vi "LED Control Module Main.vi"(8 "error in":errorcluster) -> (0 "error out":errorcluster)   [LabVIEW 2018, in "LED Control Module.lvlib"]
uses:
  LED Control Module.lvlib
  Public Controls/LVS Settings.ctl
  Public Controls/LVS Limits.ctl
  Public Controls/LVS Instruments.ctl
  Public Controls/TestData.ctl
  INI/INI File Control.ctl
  Public Controls/LVS Testplan.ctl
  Private Controls/Module Data Cluster.ctl
  Private Controls/Module Action.ctl
  <vilib>/Utility/error.llb/DialogType.ctl
  Modules/Entry Console/Entry Console/Public Controls/Entry Console.ctl
  User Events/controls/Actions.ctl
  Modules/Display Console/Display Console/public controls/Display Data.ctl
  Modules/Display Console/Display Console/Display.lvlib
  Modules/Entry Console/Entry Console/Entry Console.lvlib
  INI/LED INI File.lvlib
panel:
  in  "LED Validation":enum32{"Validation", "Settings", "Debug"}(tab)
  out "Test Visualize":cluster{dbl[], dbl[]}[](graph)=[{[0.0, 0.0, 0.0], [0.0, nan, nan]}, {[-0.05, 0.0], [0.0, 0.0]}, {[-0.05, 0.0], [0.0, 0.0]}] caption="LED Current Consumption"
  out "Messages":string
  out "History":i32(listbox)
  in  "Tester Status":string
  out "Test Status":bool=TRUE
  out "Instruments":T1 caption="LED Reference Resistors" {"Resistor 3" format="%#_g ohm"; "Resistor 2" format="%#_g ohm"; "Resistor 1" format="%#f ohm"}
  in  "Exit":bool
  in  "Logout":bool
  out "Part Number":string
  in  "Test Control":bool
  out "Clear":bool
  out "LED":bool
  out "Settings":T2 {"Source V" format="%#_g V"; "VLED 3" format="%#_g V"; "VLED 2" format="%#_g V"; "VLED 1" format="%#f V"}
  out "Limits":T3 {"Wavelength" format="%#_g nm"; "Tolerance" format="%#_g %"; "Current 3" format="%#_g  mA"; "Current 2" format="%#_g  mA"; "Current 1" format="%#_g mA"}
  in  "Role":string
  in  "Username":string
  # "LED Validation SYsTEM"
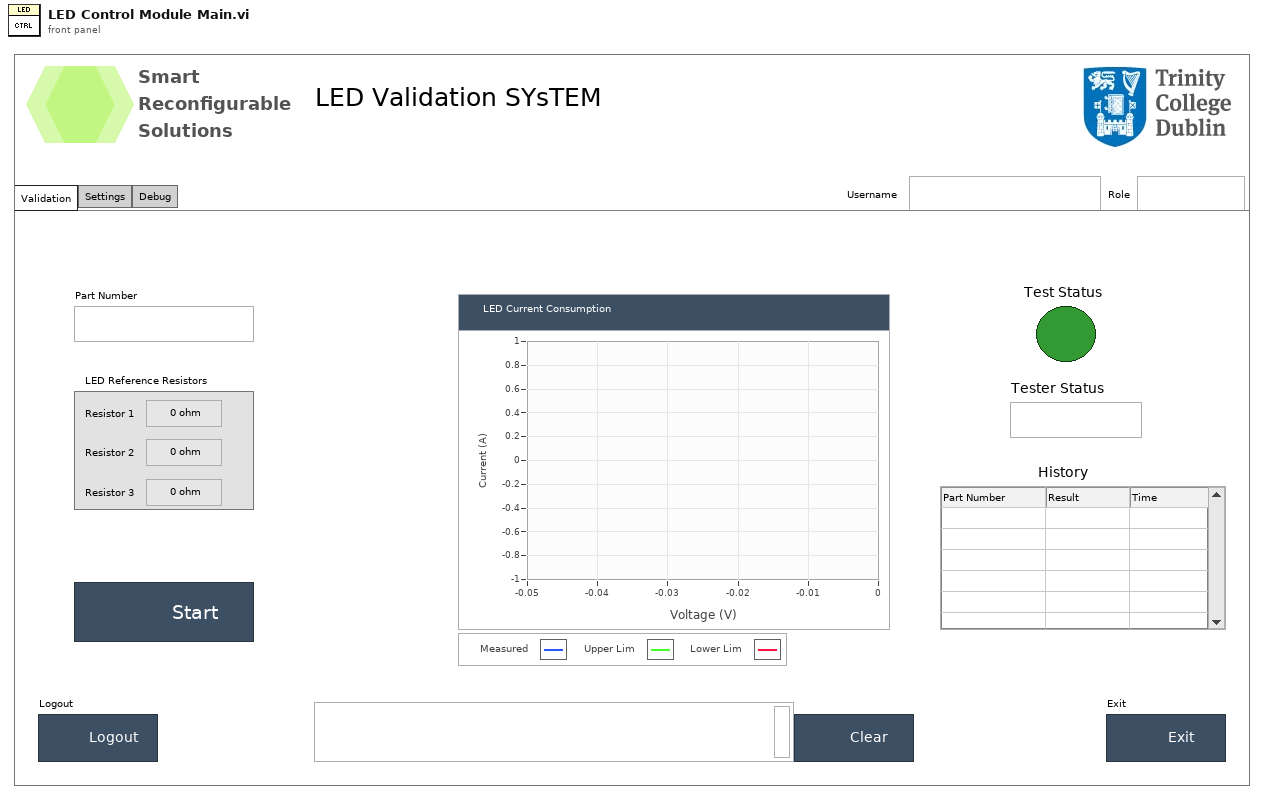
[diagram p1: front panel]
types:
  T1 = typedef "LED Control Module.lvlib/LVS Instruments.ctl" = cluster{"Resistor 1":dbl, "Resistor 2":dbl, "Resistor 3":dbl}
  T2 = typedef "LED Control Module.lvlib/LVS Settings.ctl" = cluster{"VLED 1":dbl, "VLED 2":dbl, "VLED 3":dbl, "Source V":dbl, "Result Path":path}
  T3 = typedef "LED Control Module.lvlib/LVS Limits.ctl" = cluster{"Current 1":dbl, "Current 2":dbl, "Current 3":dbl, "Tolerance":dbl, "Wavelength":dbl}
  T4 = typedef "LED Control Module.lvlib/TestData.ctl" = cluster{"data":T5, "Result Cluster":cluster{"TestResult":T6, "full date string":string, "Result":bool, "Part Number":string}}
  T5 = typedef "LED Control Module.lvlib/LED INI File.lvlib/INI File Control.ctl" = cluster{"TestPlan":T6, "Instruments":T1, "Limits":T3, "Settings":T2}
  T6 = typedef "LED Control Module.lvlib/LVS Testplan.ctl" = cluster{"Current Consumption":bool, "Emission Spectrum":bool}
  T7 = cluster{"Step Duration":string, "Station":string, "Wash Step":string}[]
  T8 = typedef "Display.lvlib/Display Data.ctl" = cluster{"Variant":variant}
  T9 = typedef "Actions.ctl" = enum16{"Get", "Create", "Destroy"}
  T10 = typedef "LED Control Module.lvlib/Module Data Cluster.ctl" = cluster{"Variant":variant, "action":T11}
  T11 = typedef "LED Control Module.lvlib/Module Action.ctl" = enum16{"init", "start", "Current", "Spectrum", "WriteResult", "---WIP---", "clear", "error", "close", "exit"}
  T12 = typedef "DialogType.ctl" = u16
  T13 = typedef "Entry Console.lvlib/Entry Console.ctl" = cluster{"Variant":variant}
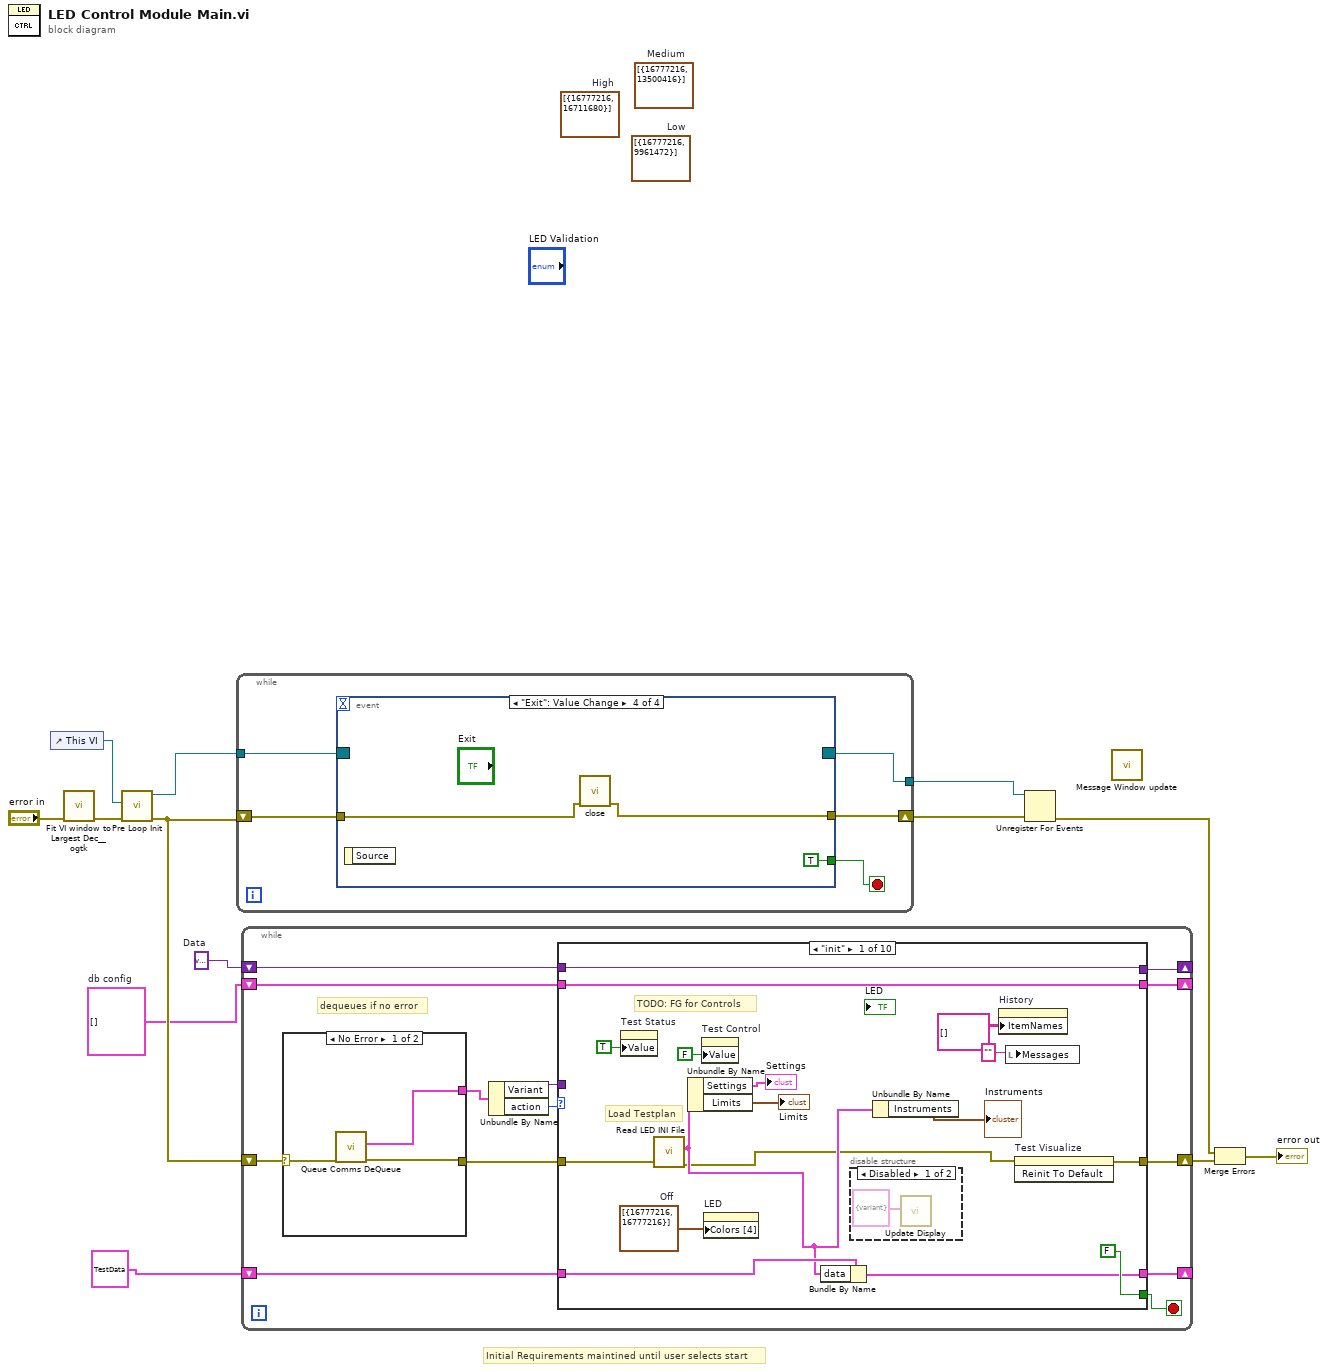
[diagram p0: block diagram]
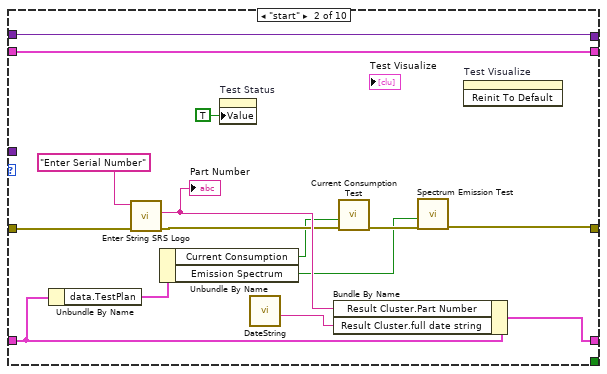
[diagram p3: hidden frame]
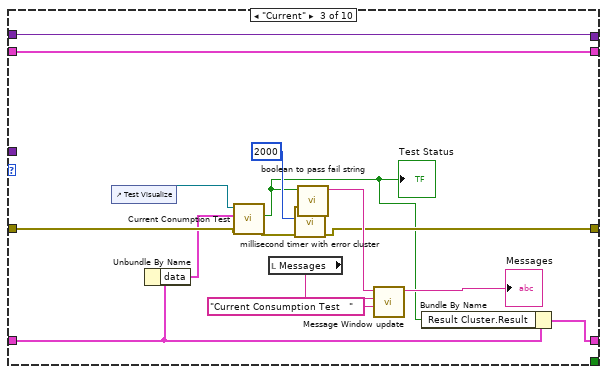
[diagram p4: hidden frame]
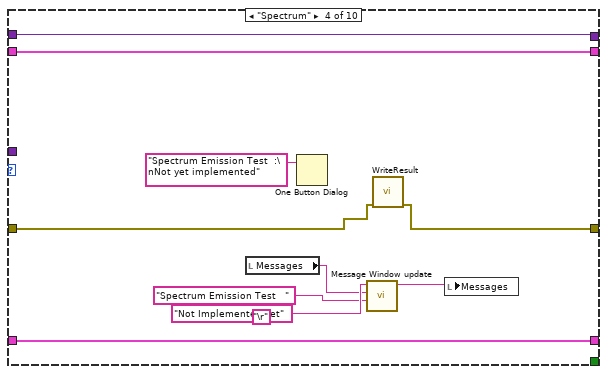
[diagram p5: hidden frame]
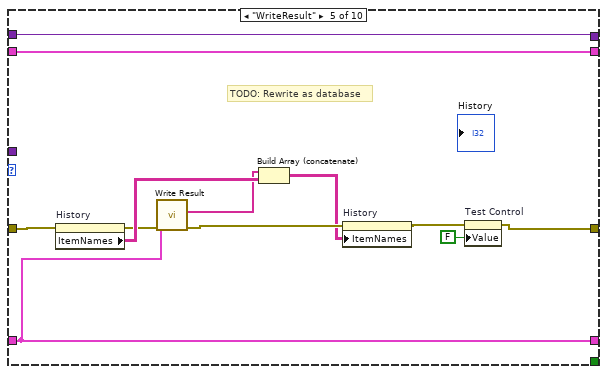
[diagram p6: hidden frame]
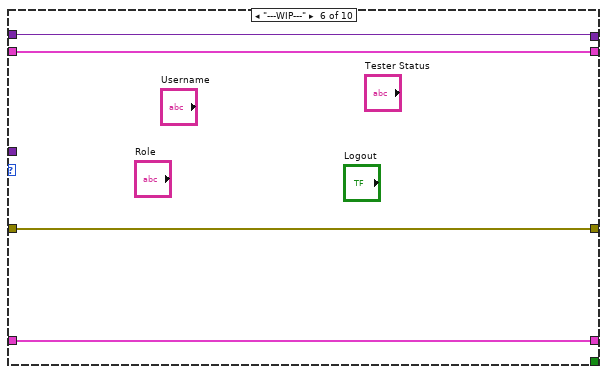
[diagram p7: hidden frame]
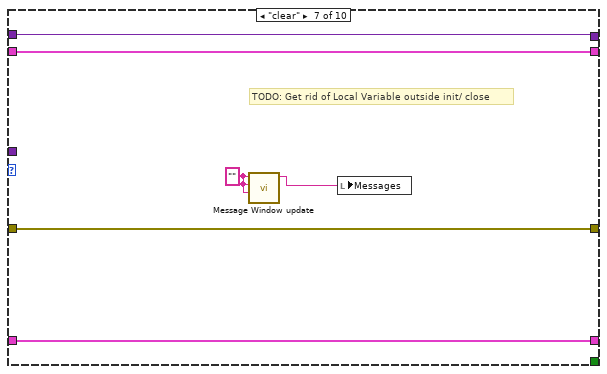
[diagram p8: hidden frame]
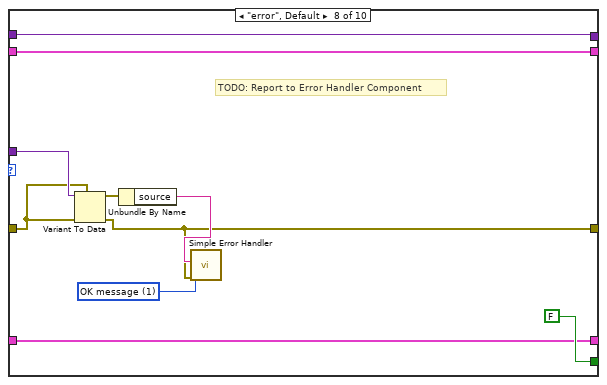
[diagram p9: hidden frame]
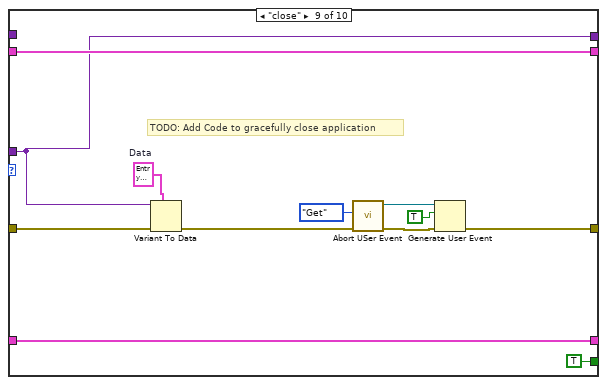
[diagram p10: hidden frame]
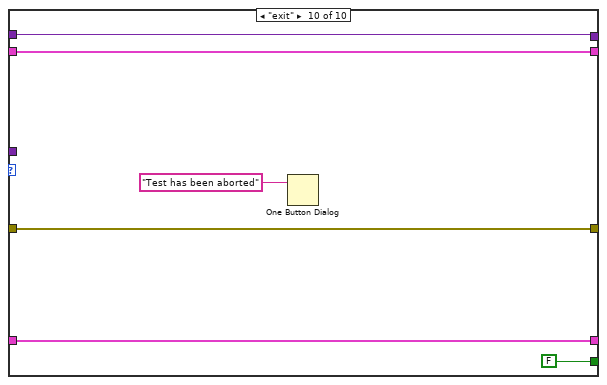
[diagram p11: hidden frame]
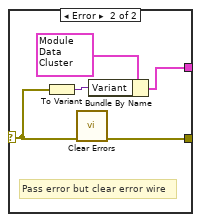
[diagram p12: hidden frame]
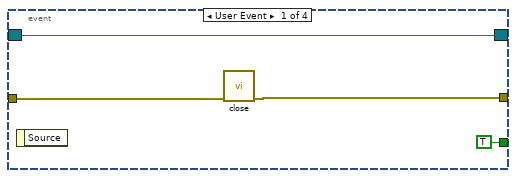
[diagram p13: hidden frame]
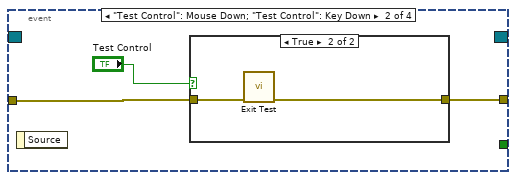
[diagram p14: hidden frame]
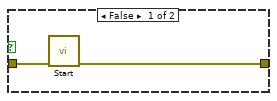
[diagram p15: hidden frame]
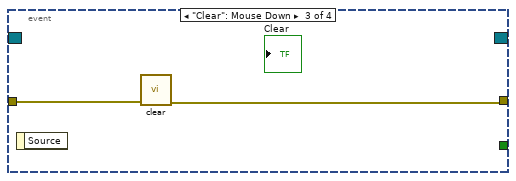
[diagram p16: hidden frame]
diagram:
  w1 = variant  # Data
  (unwired) cluster{u32, u32}[] [{16777216, 9961472}]  # Low
  (unwired) cluster{u32, u32}[] [{16777216, 13500416}]  # Medium
  (unwired) cluster{u32, u32}[] [{16777216, 16711680}]  # High
  w5 = T7 []  # db config
  # "Initial Requirements maintined until user selects start"
  n1 = control-ref of="This VI"() -> (w13:refnum<vi>)
  n2 = call <userlib>:"Fit VI window to Largest Dec__ogtk.vi"("error in (no error)"="error in") -> ("error out"=w3:errorcluster)  [unwired: 5 in, 1 out]
  n3 = call "Pre Loop Init.vi"("error in"=w3, "Ref In"=w13) -> ("error out"=w11:errorcluster, "Event Registration Refnum"=w12:refnum<event-registration>)  [unwired: 8 in]
  n4 = while {
    shift-right: [w17] -> w10
    shift-left: w11 -> [w18]
    tunnel: w12 -> [w16]
    tunnel: [w14] -> w9
    stop <- w15 stop-if-true
    n5 = event shown="[3] \"Exit\": Value Change" {
      selector: w16 -> [w19 _ _ _]
      dyn-events: [w19 _ _ _] -> w14
      timeout: _ -> [_ _ _ _]
      tunnel: w18 -> [w22 w25 w31 w34]
      tunnel: [w21 w24 w30 w33] -> w17
      tunnel: [TRUE _ _ TRUE] -> w15
      event User Event {
        n6 = event-data() -> ()  [unwired: 1 in, 1 out]
        n7 = call "close.vi"("error in"=w22) -> ("error out"=w21:errorcluster)  [unwired: 10 in]
      }
      event "Test Control": Mouse Down; "Test Control": Key Down {
        n8 = event-data() -> ()  [unwired: 1 in, 1 out]
        n9 = case shown="True" "Test Control" {
          tunnel: w25 -> [w27 w29]
          tunnel: [w26 w28] -> w24
          frame False {
            n10 = call "Start.vi"("error in"=w27) -> ("error out"=w26:errorcluster)  [unwired: 10 in]
          }
          frame True {
            n11 = call "Exit Test.vi"("error in"=w29) -> ("error out"=w28:errorcluster)  [unwired: 10 in]
          }
        }
      }
      event "Clear": Mouse Down {
        n12 = event-data() -> ()  [unwired: 1 in, 1 out]
        n13 = call "clear.vi"("error in"=w31) -> ("error out"=w30:errorcluster)  [unwired: 10 in]
      }
      event "Exit": Value Change {
        n14 = event-data() -> ()  [unwired: 1 in, 1 out]
        n15 = call "close.vi"("error in"=w34) -> ("error out"=w33:errorcluster)  [unwired: 10 in]
      }
    }
  }
  n16 = while {
    shift-right: [w44] -> w8
    shift-left: w11 -> [w47]
    shift-right: [w41] -> _
    shift-left: w5 -> [w40]
    shift-right: [w39] -> _
    shift-left: w1 -> [w38]
    shift-right: [w35] -> _
    shift-left: T4 {"data"={"TestPlan"={"Current Consumption"=TRUE, "Emission Spectrum"=TRUE}, "Instruments"={"Resistor 1"=0.0, "Resistor 2"=0.0, "Resistor 3"=0.0}, "Limits"={"Current 1"=0.0, "Current 2"=0.0, "Current 3"=0.0, "Tolerance"=0.0, "Wavelength"=0.0}, "Settings"={"VLED 1"=0.0, "VLED 2"=0.0, "VLED 3"=0.0, "Source V"=0.0, "Result Path"=path ""}}, "Result Cluster"={"TestResult"={"Current Consumption"=FALSE, "Emission Spectrum"=FALSE}, "full date string"="", "Result"=FALSE, "Part Number"=""}} ("TestData") -> [w36]
    stop <- w42 stop-if-true
    # "dequeues if no error"
    n17 = case shown="No Error" w47 {
      selector: w47 -> [w157 w162]
      tunnel: [w156 w158] -> w46
      tunnel: [w155 w161] -> w43
      frame No Error {
        n18 = call "Queue Comms DeQueue.vi"("error in"=w157) -> ("error out"=w155:errorcluster, "element"=w156:T10)  [unwired: 9 in]
      }
      frame Error {
        # "Pass error but clear error wire"
        n19 = To Variant(anything=w162) -> (Variant=w159:variant)
        n20 = call <vilib>:"Clear Errors.vi"("error in (no error)"=w162) -> ("error out"=w161:errorcluster)  [unwired: 5 in, 1 out]
        n21 = Bundle By Name(cluster=T10 {"Variant"=variant, "action"=enum."error"} ("element"), "Variant"=w159) -> (w158:T10)
      }
    }
    n22 = Unbundle By Name(w46) -> ("Variant"=w45:variant, "action"=w37:T11)
    n23 = case shown="\"init\"" w37 {
      tunnel: w45 -> [_ _ _ _ _ _ _ w132 w145 _]
      tunnel: [w48 w70 w85 w100 w106 w120 w126 w127 w139 w149] -> w44
      tunnel: w43 -> [w61 w77 w93 w101 w111 w120 w126 w131 w147 w149]
      tunnel: [FALSE _ _ _ _ _ _ FALSE TRUE FALSE] -> w42
      tunnel: [w63 w80 w95 w105 w116 w119 w125 w135 w148 w153] -> w41
      tunnel: w40 -> [w63 w80 w95 w105 w116 w119 w125 w135 w148 w153]
      tunnel: [w62 w79 w94 w104 w115 w118 w124 w134 w145 w152] -> w39
      tunnel: w38 -> [w62 w79 w94 w104 w115 w118 w124 w134 _ w152]
      tunnel: w36 -> [w60 w74 w83 w103 w114 w117 w123 w128 w146 w151]
      tunnel: [w59 w76 w81 w103 w114 w117 w123 w128 w146 w151] -> w35
      frame "init" {
        w55 = cluster{u32, u32}[] [{16777216, 16777216}]  # Off
        # "TODO: FG for Controls"
        # "Load Testplan"
        n24 = property on="Test Status" class="Bool (strict)"("Value"=TRUE ("Test Status")) -> ()  [unwired: 2 in, 2 out]
        n25 = call "Read LED INI File.vi"("error in"=w61) -> ("error out"=w49:errorcluster, "data"=w54:T5)  [unwired: 9 in]
        n26 = Unbundle By Name(w54) -> ("Settings"=→"Settings":T2, "Limits"=→"Limits":T3)
        n27 = property on="Test Control" class="Bool (strict)"("Value"=FALSE ("Test Control")) -> ()  [unwired: 2 in, 2 out]
        n28 = property on="LED" class="Bool (strict)"("Colors [4]"=w55) -> ()  [unwired: 2 in, 2 out]
        n29 = Bundle By Name(cluster=w60, "data"=w54) -> (w59:T4)
        n30 = disable-structure shown="Disabled" {
          frame Disabled {
            n31 = call "Update Display.vi"("data"=T8 {"Variant"=variant(cluster{"Variant":variant} {"Variant"=variant})} ("Cluster")) -> ()  [unwired: 10 in, 1 out]
          }
          frame Enabled {
          }
        }
        n32 = Unbundle By Name(w54) -> ("Instruments"=→"Instruments":T1)
        n33 = property on="History" class="MCListbox (strict)"("ItemNames"=string[][] [] ("Item Names")) -> ()  [unwired: 2 in, 2 out]
        n34 = local write "Messages"("" ("Messages")) -> ()
        n35 = invoke on="Test Visualize" class="XYGraph (strict)" method="Reinit To Default"(error in=w49) -> (error out=w48:errorcluster)  [unwired: 2 in, 2 out]
      }
      frame "start" {
        n36 = Unbundle By Name(w74) -> ("data.TestPlan"=w73:T6)
        n37 = call "Enter String SRS Logo.vi"("error in"=w77, "Message"="Enter Serial Number") -> ("error out"=w72:errorcluster, "String Value"=w75:string)  [unwired: 8 in]
        "Part Number" <- w75
        n38 = Unbundle By Name(w73) -> ("Current Consumption"=w69:bool, "Emission Spectrum"=w68:bool)
        n39 = property on="Test Status" class="Bool (strict)"("Value"=TRUE ("Test Status")) -> ()  [unwired: 2 in, 2 out]
        n40 = call "DateString.vi"() -> ("full date string"=w67:string)  [unwired: 7 in, 4 out]
        n41 = Bundle By Name(cluster=w74, "Result Cluster.Part Number"=w75, "Result Cluster.full date string"=w67) -> (w76:T4)
        n42 = call "Current Consumption Test.vi"("error in"=w72, "Execute"=w69) -> ("error out"=w71:errorcluster)  [unwired: 9 in]
        n43 = call "Spectrum Emission Test.vi"("error in"=w71, "Execute"=w68) -> ("error out"=w70:errorcluster)  [unwired: 9 in]
        n44 = invoke on="Test Visualize" class="XYGraph (strict)" method="Reinit To Default"() -> ()  [unwired: 3 in, 3 out]
      }
      frame "Current" {
        n45 = control-ref of="Test Visualize"() -> (w91:refnum<vi>)
        n46 = Unbundle By Name(w83) -> ("data"=w92:T5)
        n47 = call "Current Conumption Test.vi"("error in"=w93, "LED INI"=w92, "Test Visualize In"=w91) -> ("error out"=w87:errorcluster, "Pass Fail"=w82:bool)  [unwired: 6 in, 1 out]
        "Test Status" <- w82
        n48 = local read "Messages"() -> (w90:string)
        n49 = call "millisecond timer with error cluster.vi"("error in"=w87, "milliseconds to wait"=u32 2000) -> ("error out"=w85:errorcluster)  [unwired: 9 in]
        n50 = call "boolean to pass fail string.vi"("Boolean"=w82) -> ("Stat"=w89:string)  [unwired: 9 in, 1 out]
        n51 = call "Message Window update.vi"("String Control"="Current Consumption Test   ", "Previous"=w90, "Stat"=w89) -> ("String"=→"Messages":string)  [unwired: 8 in]
        n52 = Bundle By Name(cluster=w83, "Result Cluster.Result"=w82) -> (w81:T4)
      }
      frame "Spectrum" {
        (unwired) "\r"
        n53 = local read "Messages"() -> (w98:string)
        n54 = One Button Dialog(message="Spectrum Emission Test  :\nNot yet implemented") -> ()  [unwired: 1 in, 1 out]
        n55 = call "Message Window update.vi"("String Control"="Spectrum Emission Test   ", "Previous"=w98, "Stat"="Not Implemented yet" ("string")) -> ("String"=w96:string)  [unwired: 8 in]
        n56 = call "WriteResult.vi"("error in"=w101) -> ("error out"=w100:errorcluster)  [unwired: 10 in]
        n57 = local write "Messages"(w96) -> ()
      }
      frame "WriteResult" {
        # "TODO: Rewrite as database"
        n58 = property on="History" class="MCListbox (strict)"(error in=w111) -> (error out=w110:errorcluster, "ItemNames"=w113:string[][])  [unwired: 1 in, 1 out]
        n59 = call "Write Result.vi"("TestData"=w114) -> ("History Data"=w112:string[])  [unwired: 9 in, 1 out]
        n60 = Build Array (concatenate)(w112, w113) -> (w109:string[][])
        n61 = property on="History" class="MCListbox (strict)"(error in=w110, "ItemNames"=w109) -> (error out=w107:errorcluster)  [unwired: 1 in, 1 out]
        n62 = property on="Test Control" class="Bool (strict)"(error in=w107, "Value"=FALSE ("Test Control")) -> (error out=w106:errorcluster)  [unwired: 1 in, 1 out]
      }
      frame "---WIP---" {
      }
      frame "clear" {
        w122 = "" ("Stat")
        # "TODO: Get rid of Local Variable outside init/ close"
        n63 = call "Message Window update.vi"("String Control"=w122, "Previous"=w122, "Stat"=w122) -> ("String"=w121:string)  [unwired: 8 in]
        n64 = local write "Messages"(w121) -> ()
      }
      frame "error", Default {
        w133 = T12 1 items=["no dialog", "OK message", "continue or stop message", "OK message + warnings", "continue/stop + warnings"] ("type of dialog (OK msg:1)")
        # "TODO: Report to Error Handler Component"
        n65 = Variant To Data(error in=w131, type=w131, Variant=w132) -> (data=w130:errorcluster, error out=w127:errorcluster)
        n66 = Unbundle By Name(w130) -> ("source"=w129:string)
        n67 = call <vilib>:"Simple Error Handler.vi"("error source (\" \")"=w129, "type of dialog (OK msg:1)"=w133, "error in (no error)"=w127) -> ()  [unwired: 2 in, 5 out]
      }
      frame "close" {
        w144 = T13 {"Variant"=variant}  # Data
        # "TODO: Add Code to gracefully close application"
        n68 = Variant To Data(error in=w147, type=w144, Variant=w145) -> (error out=w138:errorcluster)  [unwired: 1 out]
        n69 = call "Abort USer Event.vi"("error in"=w138, "Enum"=Actions."Get") -> ("error out"=w143:errorcluster, "user event out"=w142:refnum<user-event>)  [unwired: 8 in]
        n70 = Generate User Event(user event=w142, event data cluster=TRUE ("event data"), error in=w143) -> (error out=w139:errorcluster)  [unwired: 1 in, 1 out]
      }
      frame "exit" {
        n71 = One Button Dialog(message="Test has been aborted" ("Message")) -> ()  [unwired: 1 in, 1 out]
      }
    }
  }
  n72 = Unregister For Events(event registration refnum=w9, error in=w10) -> (error out=w6:errorcluster)
  n73 = call "Message Window update.vi"() -> ()  [unwired: 11 in, 1 out]
  n74 = Merge Errors(w6, w8) -> (→"error out":errorcluster)
